vi "Get Scale UI State.vi"(8 "error in (no error)":errorcluster, 11 "references":T1) -> (0 "error out":errorcluster, 2 "active scale index":i32, 3 "scale names":string[](array[string]))   [LabVIEW 2013, in "Scaling editor node.lvclass"]
uses:
  Scaling editor node.lvclass
  <vilib>/NI/DCAF Table API/Table Manager/object ref.ctl
  <vilib>/NI/Tag Bus Data Framework/Configuration Editor/Classes/Engine Parent/Engine Parent Editor Node.lvclass
  <vilib>/NI/Tag Bus Data Framework/Configuration Editor/Classes/Module editor node/module editor node.lvclass
  module/configuration/Scaling configuration.lvclass
  module/configuration/Scaling configuration.lvclass/Scaling configuration.ctl
  Scaling editor node.lvclass/Scaling editor node.ctl
  module/configuration/accessors/Read scale names.vi
  accessors/Read active scale index .vi
  <vilib>/NI/DCAF Table API/Table Manager/Table Manager.lvclass
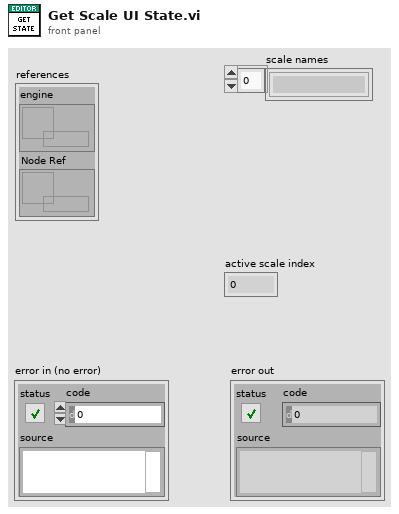
[diagram p1: front panel]
types:
  T1 = typedef "Table Manager.lvlib/Table Manager.lvclass/object ref.ctl" = cluster{"engine":refnum<data-value>, "Node Ref":refnum<data-value>}
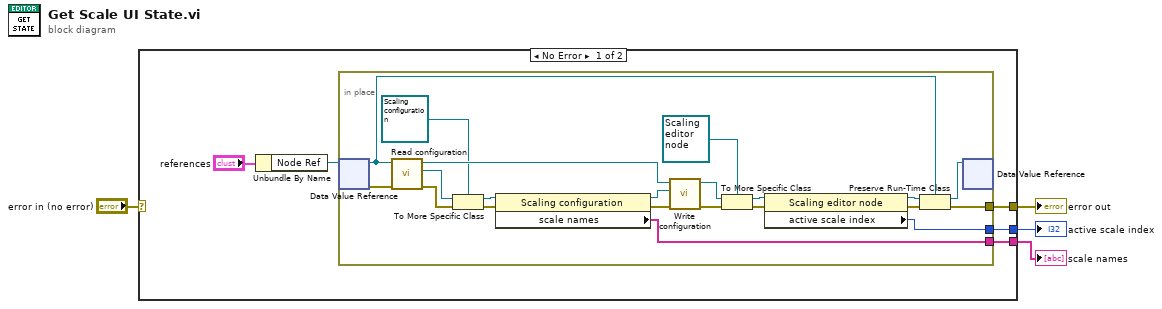
[diagram p0: block diagram]
diagram:
  n1 = case shown="No Error" "error in (no error)" {
    selector: "error in (no error)" -> [_ w31]
    tunnel: [w9 w31] -> w3
    tunnel: [w6 _] -> w2
    tunnel: [w5 _] -> w1
    frame No Error {
      n2 = Unbundle By Name("references") -> ("Node Ref"=w7:refnum<data-value>)
      n3 = in-place {
        in-place-border: [w10] -> w9
        in-place-border: [w15] -> w6
        in-place-border: [w21] -> w5
        n4 = in-place-dvr #1(w7) -> (w12:refnum<class "module editor node.lvclass">, w28:errorcluster)
        n5 = call-dynamic "Read configuration.vi"("error in"=w28, "NISE_CEF_serializable node in"=w12) -> ("error out"=w26:errorcluster, "configuration"=w29:refnum<class "NISE_CEF_serializable configuration.lvclass">, "NISE_CEF_serializable node out"=w30:refnum<class "module editor node.lvclass">)  [unwired: 7 in]
        n6 = To More Specific Class(target class=refnum<class "Scaling configuration.lvclass"> refnum ("Scaling configuration"), reference=w29, error in=w26) -> (specific class reference=w25:refnum<class "Scaling configuration.lvclass">, error out=w24:errorcluster)
        n7 = property class="Scaling configuration"(reference=w25, error in=w24) -> (reference out=w23:refnum<class "Scaling configuration.lvclass">, error out=w22:errorcluster, "scale names"=w21:string[])
        n8 = call-dynamic "Write configuration.vi"("error in"=w22, "configuration"=w23, "NISE_CEF_serializable node in"=w30) -> ("error out"=w19:errorcluster, "NISE_CEF_serializable node out"=w20:refnum<class "module editor node.lvclass">)  [unwired: 7 in]
        n9 = To More Specific Class(target class=refnum<class "Scaling editor node.lvclass"> refnum ("Scaling editor node"), reference=w20, error in=w19) -> (specific class reference=w17:refnum<class "Scaling editor node.lvclass">, error out=w16:errorcluster)
        n10 = property class="Scaling editor node"(reference=w17, error in=w16) -> (reference out=w13:refnum<class "Scaling editor node.lvclass">, error out=w14:errorcluster, "active scale index "=w15:i32)
        n11 = Preserve Run-Time Class(object in=w13, error in=w14, 2:w12) -> (object out=w11:refnum<class "module editor node.lvclass">, error out=w10:errorcluster)
        n12 = in-place-dvr #1(w11) -> ()  [unwired: 2 out]
      }
    }
    frame Error {
    }
  }
  "error out" <- w3
  "active scale index" <- w2
  "scale names" <- w1
